vi "AO Activate.vi"(7 "AO Task":refnum<k21>, 8 "error constant":errorcluster, 10 "AO":T1(array[cluster])) -> (0 "error out":errorcluster, 3 "Abort":bool)   [LabVIEW 2022 SP3]
uses:
  RT Controls/AO FGV.ctl
  <vilib>/DAQmx/write.llb/DAQmx Write (Analog 1D DBL NChan 1Samp).vi
  RT Sub VI's/RT Global.vi
  <vilib>/DAQmx/miscellaneous.llb/DAQmx Fill In Error Info.vi
panel:
  out "Seq State":string
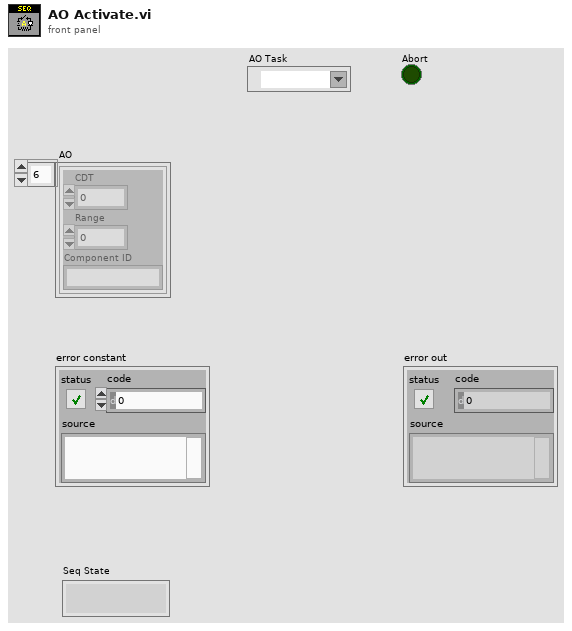
[diagram p1: front panel]
types:
  T1 = cluster{"CDT":dbl, "Range":dbl, "Component ID":string}[]
  T2 = cluster{"AO":cluster{"CDT":dbl, "Range":dbl, "Component ID":string}[], "DO":cluster{"CDT":dbl, "Position":bool, "Component ID":string}[], "Launch Time":timestamp}
  T3 = typedef "AO FGV.ctl" = enum16{"Read", "Write", "Start time", "init", "Read Only"}
  T4 = cluster{"CDT":dbl, "Range":dbl, "Component ID":string}
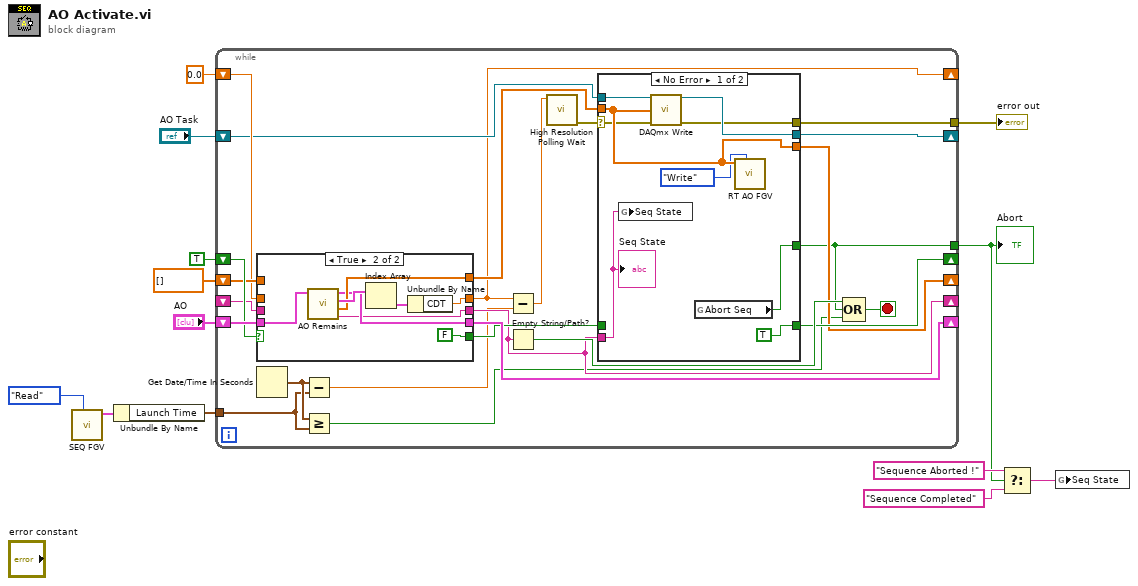
[diagram p0: block diagram]
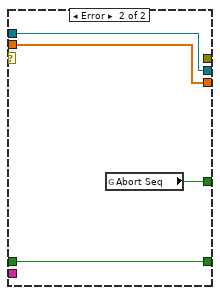
[diagram p2: hidden frame]
diagram:
  n1 = call "SEQ FGV.vi"("Enum"=enum16{"Read", "Write"}."Read") -> ("Seq data out"=w11:T2)  [unwired: 9 in, 1 out]
  n2 = Unbundle By Name(w11) -> ("Launch Time"=w5:timestamp)
  n3 = while {
    shift-right: [w29] -> _
    shift-left: "AO" -> [w37]
    shift-right: [w26] -> _
    shift-left: TRUE -> [w36]
    shift-right: [w25] -> _
    shift-left: dbl[] [] ("DO value") -> [w35]
    shift-right: [w19] -> _
    shift-left: 0.0 ("CDT") -> [w34]
    shift-right: [w31] -> _
    shift-left: "AO Task" -> [w32]
    tunnel: w5 -> [w21]
    shift-right: [w23] -> _
    shift-left: _ -> [w24]
    tunnel: [w15] -> w2
    tunnel: [w14] -> w1
    stop <- w30 stop-if-true
    n4 = case shown="True" w36 {
      selector: w36 -> [w52 _]
      tunnel: w37 -> [w53 w63]
      tunnel: [w53 w58] -> w29
      tunnel: [w55 w60] -> w33
      tunnel: w35 -> [w55 _]
      tunnel: [w54 w59] -> w19
      tunnel: w34 -> [w54 _]
      tunnel: [w52 FALSE] -> w27
      tunnel: [w51 w56] -> w23
      tunnel: w24 -> [w51 _]
      frame False {
      }
      frame True {
        n5 = call "AO Remains.vi"("Array"=w63) -> ("String"=w56:string, "AO"=w60:dbl[], "Same AO"=w62:T1, "Remains AO"=w58:T1)  [unwired: 7 in]
        n6 = Index Array(array=w62) -> (element=w61:T4)  [unwired: 1 in]
        n7 = Unbundle By Name(w61) -> ("CDT"=w59:dbl)
      }
    }
    n8 = Get Date/Time In Seconds() -> (seconds since 1Jan1904=w22:timestamp)
    n9 = Subtract(x=w22, y=w21) -> (x-y=w18:dbl)
    n10 = Greater Or Equal?(x=w22, y=w21) -> (x >= y?=w20:bool)
    n11 = Subtract(x=w19, y=w18) -> (x-y=w17:dbl)
    n12 = Empty String/Path?(string/path=w23) -> (empty?=w28:bool)
    n13 = call <vilib>:"High Resolution Polling Wait.vi"("seconds to wait"=w17) -> ("error out"=w16:errorcluster)  [unwired: 10 in]
    n14 = case shown="No Error" w16 {
      selector: w16 -> [w41 _]
      tunnel: w33 -> [w42 w50]
      tunnel: [w42 w50] -> w25
      tunnel: w32 -> [w46 w49]
      tunnel: [w45 w49] -> w31
      tunnel: [w44 _] -> w15
      tunnel: w27 -> [_ w48]
      tunnel: [TRUE w48] -> w26
      tunnel: w23 -> [w38 _]
      tunnel: [w39 w47] -> w14
      frame No Error {
        n15 = global write "RT Global.vi" "Seq State"(w38) -> ()
        n16 = call-poly <vilib>:"DAQmx Write.vi"("task/channels in"=w46, "data"=w42, "error in"=w41) -> ("task out"=w45:refnum<k21>, "error out"=w44:errorcluster)  [unwired: 10 in, 1 out]
        n17 = global read "RT Global.vi" "Abort Seq"() -> (w39:bool)
        n18 = call "RT AO FGV.vi"("Enum"=AO_FGV."Write", "AO in"=w42) -> ()  [unwired: 7 in, 3 out]
        "Seq State" <- w38
      }
      frame Error {
        n19 = global read "RT Global.vi" "Abort Seq"() -> (w47:bool)
      }
    }
    n20 = Compound Arithmetic op=OR(w28, w14, w20) -> (w30:bool)
  }
  "error out" <- w2
  "Abort" <- w1
  n21 = Select(t="Sequence Aborted !" ("Seq State"), s=w1, f="Sequence Completed" ("Seq State")) -> (s? t:f=w6:string)
  n22 = global write "RT Global.vi" "Seq State"(w6) -> ()
